vi "fs_mm_converter.vi"(2 "mm in":dbl, 3 "fs in":dbl) -> (0 "mm out":dbl, 1 "fs out":dbl)   [LabVIEW 2019, in "smc100.lvlib"]
uses:
  smc100.lvlib
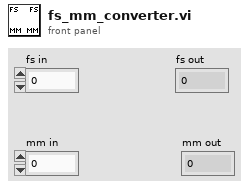
[diagram p1: front panel]
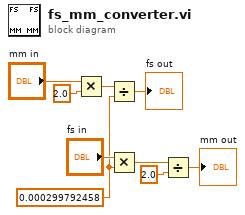
[diagram p0: block diagram]
diagram:
  w1 = 0.000299792458 ("y")
  n1 = Multiply(x="mm in", y=2.0) -> (x*y=w7:dbl)
  n2 = Divide(x=w7, y=w1) -> (x/y=→"fs out":dbl)
  n3 = Multiply(x="fs in", y=w1) -> (x*y=w5:dbl)
  n4 = Divide(x=w5, y=2.0) -> (x/y=→"mm out":dbl)
